vi "Select Actor Dialog.vi"(8 "Error In":errorcluster, 11 "CS++ObjectManager":refnum<class "CS++ObjectManager.lvclass">) -> (0 "Error Out":errorcluster, 2 "Selected Names":string[](array[string]), 3 "CS++ObjectManager":refnum<class "CS++ObjectManager.lvclass">)   [LabVIEW 2016, in "CS++ObjectManager.lvlib" / "CS++ObjectManager.lvclass"]
doc: "Read Actor List from DB and display selection dialog."
uses:
  CS++ObjectManager.lvclass
  CS++ObjectManager.lvclass/CS++ObjectManager.ctl
panel:
  in  "Actor List":i32[](listbox)
  in  "Cancel":bool
  in  "Launch":bool
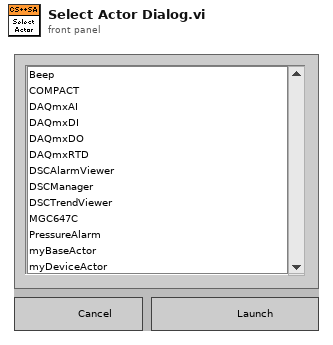
[diagram p1: front panel]
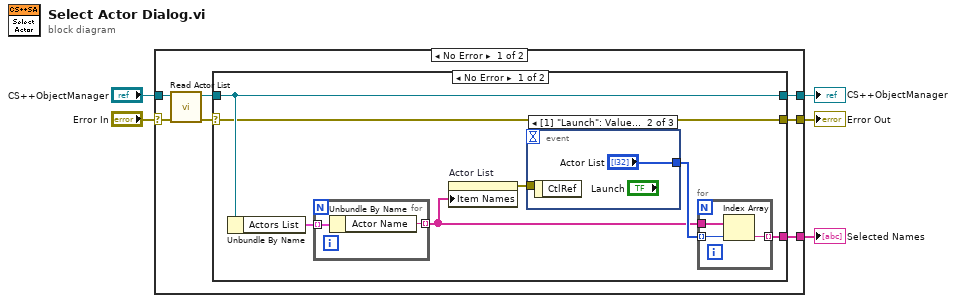
[diagram p0: block diagram]
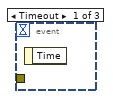
[diagram p2: hidden frame]
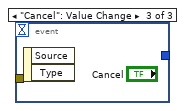
[diagram p3: hidden frame]
diagram:
  n1 = case shown="No Error" "Error In" {
    selector: "Error In" -> [w7 w28]
    tunnel: [w12 _] -> w5
    tunnel: "CS++ObjectManager" -> [w9 w29]
    tunnel: [w11 w29] -> w3
    tunnel: [w10 w28] -> w1
    frame No Error {
      n2 = call "Read Actor List.vi"("error in (no error)"=w7, "CS++ObjectManager in"=w9) -> ("error out"=w6:errorcluster, "CS++ObjectManager out"=w8:refnum<class "CS++ObjectManager.lvclass">)  [unwired: 8 in]
      n3 = case shown="No Error" w6 {
        selector: w6 -> [w13 w26]
        tunnel: [w17 _] -> w12
        tunnel: w8 -> [w14 w27]
        tunnel: [w14 w27] -> w11
        tunnel: [w13 w26] -> w10
        frame No Error {
          n4 = Unbundle By Name(w14) -> ("Actors List"=w15:cluster{"Actor Name":string, "Open":bool}[])
          n5 = for {
            tunnel: w15 -> [w21] mode=indexing
            tunnel: [w20] -> w16 mode=indexing
            n6 = Unbundle By Name(w21) -> ("Actor Name"=w20:string)
          }
          n7 = property on="Actor List" class="LstBox (strict)"("Item Names"=w16) -> (error out=w19:errorcluster)  [unwired: 2 in, 1 out]
          n8 = event shown="[1] \"Launch\": Value Change;  \"Actor List\": Double Click" {
            selector: _ -> [_ _ _]
            dyn-events: _ -> [_ _ _]
            timeout: _ -> [_ _ _]
            tunnel: [_ "Actor List" _] -> w18
            tunnel: w19 -> [_ _ _]
            event Timeout {
              n9 = event-data() -> ()  [unwired: 1 in, 1 out]
            }
            event "Launch": Value Change; "Actor List": Double Click {
              n10 = event-data() -> ()  [unwired: 1 in, 1 out]
            }
            event "Cancel": Value Change {
              n11 = event-data() -> ()  [unwired: 1 in, 2 out]
            }
          }
          n12 = for {
            tunnel: w18 -> [w23] mode=indexing
            tunnel: w16 -> [w24]
            tunnel: [w22] -> w17 mode=indexing
            n13 = Index Array(array=w24, index=w23) -> (element=w22:string)
          }
        }
        frame Error {
        }
      }
    }
    frame Error {
    }
  }
  "Selected Names" <- w5
  "CS++ObjectManager" <- w3
  "Error Out" <- w1
